vi "Initialize.vi"(7 "Serial Configuration":T1={"Baud Rate"=9600, "Parity"=2, "Data Bits"=7} {"Data Bits" items=["7"=7, "8"=8]; "Parity" items=["None", "Odd", "Even"]; "Baud Rate" items=["300"=300, "600"=600, "1200"=1200, "2400"=2400, "4800"=4800, "9600"=9600, "19200"=19200]}, 8 "error in (no error)":errorcluster, 9 "Reset (True)":bool=TRUE, 10 "ID Query (True)":bool=TRUE, 11 "VISA resource name":refnum<visa-resource-name>) -> (0 "error out":errorcluster, 2 "id":string, 3 "VISA resource name out":refnum<visa-resource-name>)   [LabVIEW 2011, in "Agilent 34401.lvlib"]
doc: "Establishes communication with the instrument and optionally performs an instrument identification query and/or an instrument reset. It also places the instrument in a default state needed for other instrument driver operations. Therefore, call this VI before calling other instrument driver VIs for this instrument. Generally, you need to call the <B>Initialize VI</B> only once at the beginning of an application."
uses:
  Agilent 34401.lvlib
  Private/Extended User Data.ctl
panel:
  # "(c) 2005-2008 National Instruments.  ALL RIGHTS RESERVED."
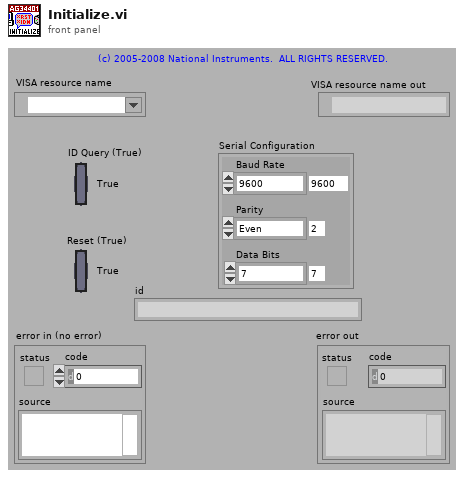
[diagram p1: front panel]
types:
  T1 = cluster{"Baud Rate":u32, "Parity":u16, "Data Bits":u16}
  T2 = typedef "Agilent 34401.lvlib/Extended User Data.ctl" = cluster{"Trigger Source":u16, "Math Storage":u16, "Agilent Model":i32}
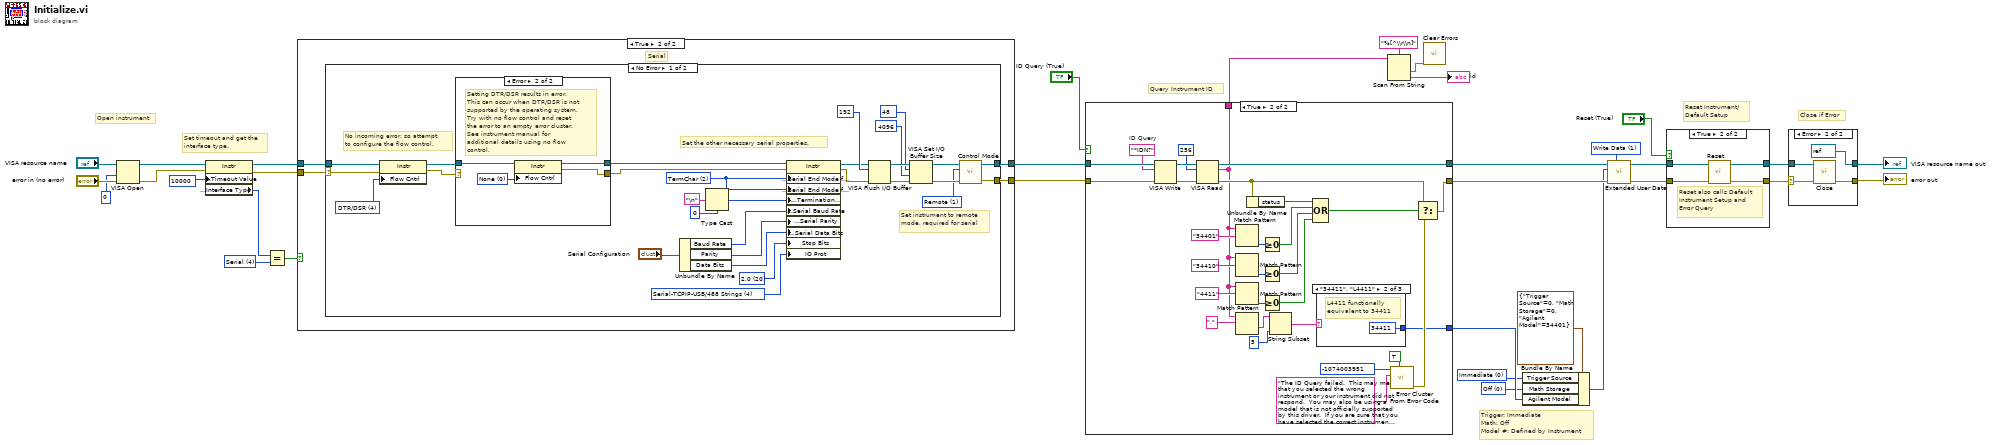
[diagram p0: block diagram]
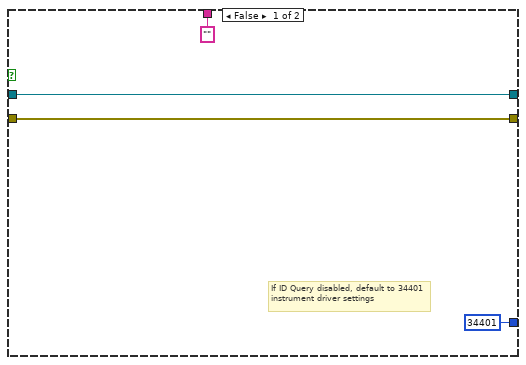
[diagram p2: hidden frame]
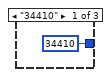
[diagram p3: hidden frame]
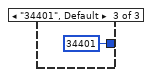
[diagram p4: hidden frame]
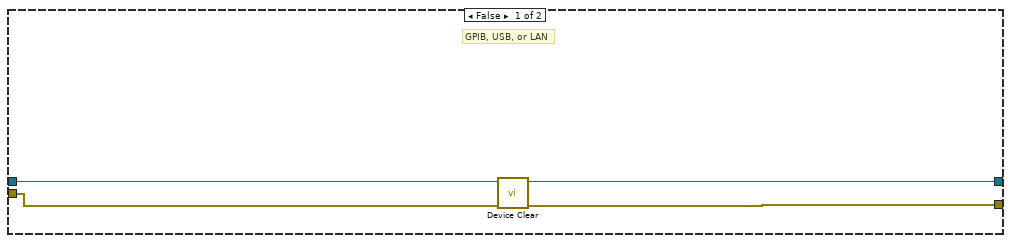
[diagram p5: hidden frame]
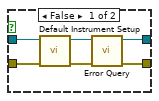
[diagram p9: hidden frame]
diagram:
  w6 = u16 0 items=["Immediate", "Software (Bus)", "External", "Internal"] ("Trigger Source")
  w7 = u16 0 items=["Off", "Internal Buffer", "Output Buffer"] ("Math Storage")
  w10 = u16 1 items=["Read Data", "Write Data", "Dispose of Data"] ("Action")
  w27 = u16 4 items=["GPIB"=1, "VXI"=2, "GPIB-VXI"=3, "Serial"=4, "PXI"=5, "TCPIP"=6, "USB"=7] ("Interface Information:Interface Type")
  # "Trigger: Immediate\nMath: Off\nModel #: Defined by Instrument"
  # "Set timeout and get the\ninterface type."
  # "Close if Error"
  # "Query Instrument ID"
  # "Reset Instrument/\nDefault Setup"
  # "Open instrument"
  n1 = VISA Open(access mode=u32 0, error in (no error)="error in (no error)", VISA resource name="VISA resource name") -> (VISA resource name=w18:refnum<visa-resource-name>, error out=w17:errorcluster)  [unwired: 2 in]
  n2 = property on="Property Node" class="Instr"(reference=w18, error in=w17, "General Settings:Timeout Value"=u32 10000) -> (reference out=w16:refnum<visa-resource-name>, error out=w15:errorcluster, "Interface Information:Interface Type"=w30:u16)
  n3 = Equal?(x=w30, y=w27) -> (x = y?=w28:bool)
  n4 = case shown="True" w28 {
    tunnel: [w35 w41] -> w21
    tunnel: [w34 w40] -> w19
    tunnel: w16 -> [w36 w39]
    tunnel: w15 -> [w37 w38]
    frame False {
      # "GPIB, USB, or LAN"
      n5 = call "Device Clear.vi"("error in (no error)"=w37, "VISA Resource Name"=w36) -> ("error out"=w34:errorcluster, "VISA Resource Out"=w35:refnum<visa-resource-name>)  [unwired: 8 in]
    }
    frame True {
      # "Serial"
      n6 = case shown="No Error" w38 {
        selector: w38 -> [w42 w77]
        tunnel: [w63 w78] -> w41
        tunnel: [w62 w77] -> w40
        tunnel: w39 -> [w59 w78]
        frame No Error {
          w56 = u16 4 items=["Normal"=1, "VXI/FDC"=2, "GPIB/HS488"=3, "Serial-TCPIP-USB/488 Strings"=4, "USBTMC/Vendor-Specific"=5] ("Message Based Settings:IO Protocol")
          w55 = u16 20 items=["1.0"=10, "1.5"=15, "2.0"=20] ("Serial Settings:Serial Stop Bits")
          w49 = u16 2 items=["None", "LastBit", "TermChar"] ("Serial Settings:Serial End Mode for Reads")
          w61 = u16 1 items=["Local", "Remote", "Remote with Lock"] ("Control Mode (0:Local)")
          w60 = u16 4 items=["None", "XON/XOFF", "RTS/CTS", "XON/XOFF & RTS/CTS", "DTR/DSR", "XON/XOFF & DTR/DSR"] ("Serial Settings:Serial Flow Control")
          # "Set the other necessary serial properties."
          # "No incoming error, so attempt to configure the flow control."
          # "Set instrument to remote mode, required for serial"
          n7 = property on="Property Node" class="Instr"(reference=w59, error in=w42, "Flow Cntrl"=w60) -> (reference out=w58:refnum<visa-resource-name>, error out=w57:errorcluster)
          n8 = case shown="Error" w57 {
            selector: w57 -> [w71 _]
            tunnel: w58 -> [w72 w73]
            tunnel: [w72 w74] -> w45
            tunnel: [w71 w75] -> w46
            frame No Error {
              # "Setting DTR/DSR flow control successful so proceed."
            }
            frame Error {
              w76 = u16 0 items=["None", "XON/XOFF", "RTS/CTS", "XON/XOFF & RTS/CTS", "DTR/DSR", "XON/XOFF & DTR/DSR"] ("Serial Settings:Serial Flow Control")
              # "Setting DTR/DSR results in error. This can occur when DTR/DSR is not supported by the operating system.  Try with no flow control and reset the error to an empty error cluster. See instrument manual for additional details using no flow control."
              n9 = property on="Property Node" class="Instr"(reference=w73, "Flow Cntrl"=w76) -> (reference out=w74:refnum<visa-resource-name>, error out=w75:errorcluster)  [unwired: 1 in]
            }
          }
          n10 = Unbundle By Name("Serial Configuration") -> ("Baud Rate"=w52:u32, "Parity"=w54:u16, "Data Bits"=w53:u16)
          n11 = Type Cast(type=u8 0, x="\n" ("Line Feed Constant")) -> (*(type *) &x=w50:u8)
          n12 = property on="Property Node" class="Instr"(reference=w45, error in=w46, "Serial Settings:Serial End Mode for Reads"=w49, "Serial Settings:Serial End Mode for Writes"=w49, "Message Based Settings:Termination Character"=w50, "Serial Settings:Serial Baud Rate"=w52, "Serial Settings:Serial Parity"=w54, "Serial Settings:Serial Data Bits"=w53, "Stop Bits"=w55, "IO Prot"=w56) -> (reference out=w44:refnum<visa-resource-name>, error out=w43:errorcluster)
          n13 = VISA Flush I/O Buffer(VISA resource name=w44, mask (16)=u16 192, error in (no error)=w43) -> (VISA resource name out=w70:refnum<visa-resource-name>, error out=w69:errorcluster)
          n14 = VISA Set I/O Buffer Size(VISA resource name=w70, mask (16)=u16 48, size (4096)=u32 4096 ("size (0)"), error in (no error)=w69) -> (VISA resource name out=w65:refnum<visa-resource-name>, error out=w64:errorcluster)
          n15 = call "Control Mode.vi"("error in (no error)"=w64, "Control Mode (0:Local)"=w61, "VISA Resource Name"=w65) -> ("error out"=w62:errorcluster, "VISA Resource Out"=w63:refnum<visa-resource-name>)  [unwired: 7 in]
        }
        frame Error {
          # "If there is an error in, do not attempt to set additional serial parameters."
        }
      }
    }
  }
  n16 = case shown="True" "ID Query (True)" {
    tunnel: [w81 w112] -> w13
    tunnel: [w82 w109] -> w12
    tunnel: w21 -> [w82 w110]
    tunnel: w19 -> [w81 w111]
    tunnel: [34401 w84] -> w8
    tunnel: ["" ("read buffer") w83] -> w4
    frame False {
      # "If ID Query disabled, default to 34401 instrument driver settings"
    }
    frame True {
      w104 = "*IDN?"  # ID Query
      n17 = VISA Write(VISA resource name=w110, write buffer=w104, error in (no error)=w111) -> (VISA resource name out=w108:refnum<visa-resource-name>, error out=w107:errorcluster)  [unwired: 1 out]
      n18 = VISA Read(VISA resource name=w108, byte count=u32 256, error in (no error)=w107) -> (VISA resource name out=w109:refnum<visa-resource-name>, read buffer=w83:string, error out=w98:errorcluster)  [unwired: 1 out]
      n19 = Match Pattern(string=w83, regular expression="34401") -> (offset past match=w99:i32)  [unwired: 1 in, 3 out]
      n20 = Match Pattern(string=w83, regular expression="34410") -> (offset past match=w96:i32)  [unwired: 1 in, 3 out]
      n21 = Match Pattern(string=w83, regular expression="4411") -> (offset past match=w95:i32)  [unwired: 1 in, 3 out]
      n22 = Match Pattern(string=w83, regular expression=",") -> (after substring=w87:string)  [unwired: 1 in, 3 out]
      n23 = Unbundle By Name(w98) -> ("status"=w97:bool)
      n24 = Greater Or Equal To 0?(x=w99) -> (x >= 0?=w92:bool)
      n25 = Greater Or Equal To 0?(x=w96) -> (x >= 0?=w91:bool)
      n26 = Greater Or Equal To 0?(x=w95) -> (x >= 0?=w90:bool)
      n27 = String Subset(string=w87, length (rest)=5 ("length (rest)")) -> (substring=w85:string)  [unwired: 1 in]
      n28 = Compound Arithmetic op=OR(w97, w92, w91, w90) -> (w89:bool)
      n29 = case shown="\"34411\", \"L4411\"" w85 {
        tunnel: [34410 ("number 3") 34411 ("number 3") 34401 ("number 3")] -> w84
        frame "34410" {
        }
        frame "34411", "L4411" {
          # "L4411 functionally equivalent to 34411"
        }
        frame "34401", Default {
        }
      }
      n30 = call <vilib>:"Error Cluster From Error Code.vi"("show call chain? (False)"=TRUE, "error message (\"\")"="The ID Query failed.  This may mean that you selected the wrong instrument or your instrument did not respond.  You may also be using a model that is not officially supported by this driver.  If you are sure that you have selected the correct instrument and it is responding, try disabling the ID Query." ("Source (VI Name)"), "error code (0)"=-1074003951 ("Code")) -> ("error out"=w103:errorcluster)  [unwired: 6 in]
      n31 = Select(t=w98, s=w89, f=w103) -> (s? t:f=w112:errorcluster)
    }
  }
  n32 = Scan From String(format string="%[^\\r\\n]", input string=w4) -> (error out=w1:errorcluster, output 1=→"id":string)  [unwired: 3 in, 2 out]
  n33 = call <vilib>:"Clear Errors.vi"("error in (no error)"=w1) -> ()  [unwired: 6 in, 1 out]
  n34 = Bundle By Name(cluster=T2 {"Trigger Source"=0, "Math Storage"=0, "Agilent Model"=34401} ("User Data Definition"), "Trigger Source"=w6, "Math Storage"=w7, "Agilent Model"=w8) -> (w5:T2)
  n35 = call "Extended User Data.vi"("Action"=w10, "Error In (no error)"=w13, "User Data In"=w5, "VISA resource name in"=w12) -> ("Error Out"=w14:errorcluster, "VISA resource name out"=w11:refnum<visa-resource-name>)  [unwired: 5 in, 1 out]
  n36 = case shown="True" "Reset (True)" {
    tunnel: w14 -> [w120 w122]
    tunnel: [w117 w125] -> w23
    tunnel: w11 -> [w121 w123]
    tunnel: [w116 w124] -> w24
    frame False {
      n37 = call "Default Instrument Setup.vi"("error in (no error)"=w120, "VISA resource name"=w121) -> ("error out"=w118:errorcluster, "VISA resource name out"=w119:refnum<visa-resource-name>)  [unwired: 8 in]
      n38 = call "Error Query.vi"("error in (no error)"=w118, "VISA resource name"=w119) -> ("error out"=w117:errorcluster, "VISA resource name out"=w116:refnum<visa-resource-name>)  [unwired: 6 in, 2 out]
    }
    frame True {
      # "Reset also calls Default Instrument Setup and Error Query"
      n39 = call "Reset.vi"("error in (no error)"=w122, "VISA resource name"=w123) -> ("error out"=w125:errorcluster, "VISA resource name out"=w124:refnum<visa-resource-name>)  [unwired: 8 in]
    }
  }
  n40 = case shown="Error" w23 {
    selector: w23 -> [w126 w129]
    tunnel: w24 -> [w127 w130]
    tunnel: [w127 refnum<visa-resource-name> refnum ("VISA resource name out")] -> w25
    tunnel: [w126 w131] -> w20
    frame No Error {
    }
    frame Error {
      n41 = call "Close.vi"("error in (no error)"=w129, "VISA resource name"=w130) -> ("error out"=w131:errorcluster)  [unwired: 9 in]
    }
  }
  "VISA resource name out" <- w25
  "error out" <- w20
